vi "LD-Cal-CircleCenterXY -矩形.vi"(0 "Image in":T5(plugin-control), 5 "String":string=";1480.000;1115.000;378.000;757.000;0.000;0.000;0;1;3;3;10.000;4;0;1;0;0;1;65280;255;16776960;16711680;;3;10;3;23;255", 11 "error in":errorcluster) -> (4 "Image Out":T5(plugin-control), 6 "Straight Edge (Find Straight Edge 2)":T4 {"Point2 (Real-World)"."Y" format="%.2f"; "Point2 (Real-World)"."X" format="%.2f"; "Point1 (Real-World)"."Y" format="%.2f"; "Point1 (Real-World)"."X" format="%.2f"; "Point2 (Pixels)"."Y" format="%.2f"; "Point2 (Pixels)"."X" format="%.2f"; "Point1 (Pixels)"."Y" format="%.2f"; "Point1 (Pixels)"."X" format="%.2f"}, 8 "Angle (Pixel)":dbl, 10 "result string":string, 15 "error out":errorcluster)   [LabVIEW 2015]
uses:
  <vilib>/vision/Measure.llb/Edge Options.ctl
  <vilib>/vision/Measure.llb/Edge Polarity.ctl
  <vilib>/vision/Measure.llb/Straight Edge Options.ctl
  <vilib>/vision/Measure.llb/Straight Edge Process.ctl
panel:
  out "Angle (Pixel) 3":dbl
  in  "Options (Find Straight Edge 2)":T3={"Search Direction"=2, "Edge Options"={"Edge Polarity"=2, "Kernel Size"=5, "Width"=11, "Minimum Edge Strength"=76.237114, "Interpolation Type"=enum."Bilinear Fixed", "Data Processing Method"=enum."Average"}, "Show Search Area"=TRUE, "Show Search Lines"=TRUE, "Show Edges Found"=TRUE, "Show Result"=TRUE, "Search Area Color"=65280, "Search Lines Color"=255, "Edge Locations Color"=16776960, "Result Color"=16711680, "Overlay Group Name"=""} {"Search Direction" items=["Left to Right", "Right to Left", "Top to Bottom", "Bottom to Top"]; "Edge Options"."Edge Polarity" items=["All Edges", "Rising Edges", "Falling Edges"]; "Edge Options"."Minimum Edge Strength" format="%.2f"; "Edge Options"."Width" step=2; "Edge Options"."Kernel Size" step=2}
  in  "Option All":T3 {"Edge Options"."Edge Polarity" items=["All Edges", "Rising Edges", "Falling Edges"]; "Edge Options"."Minimum Edge Strength" format="%.2f"; "Edge Options"."Width" step=2; "Edge Options"."Kernel Size" step=2}
  out "Center (Pixels)":cluster{"X":string, "Y":string, "Radius":string}
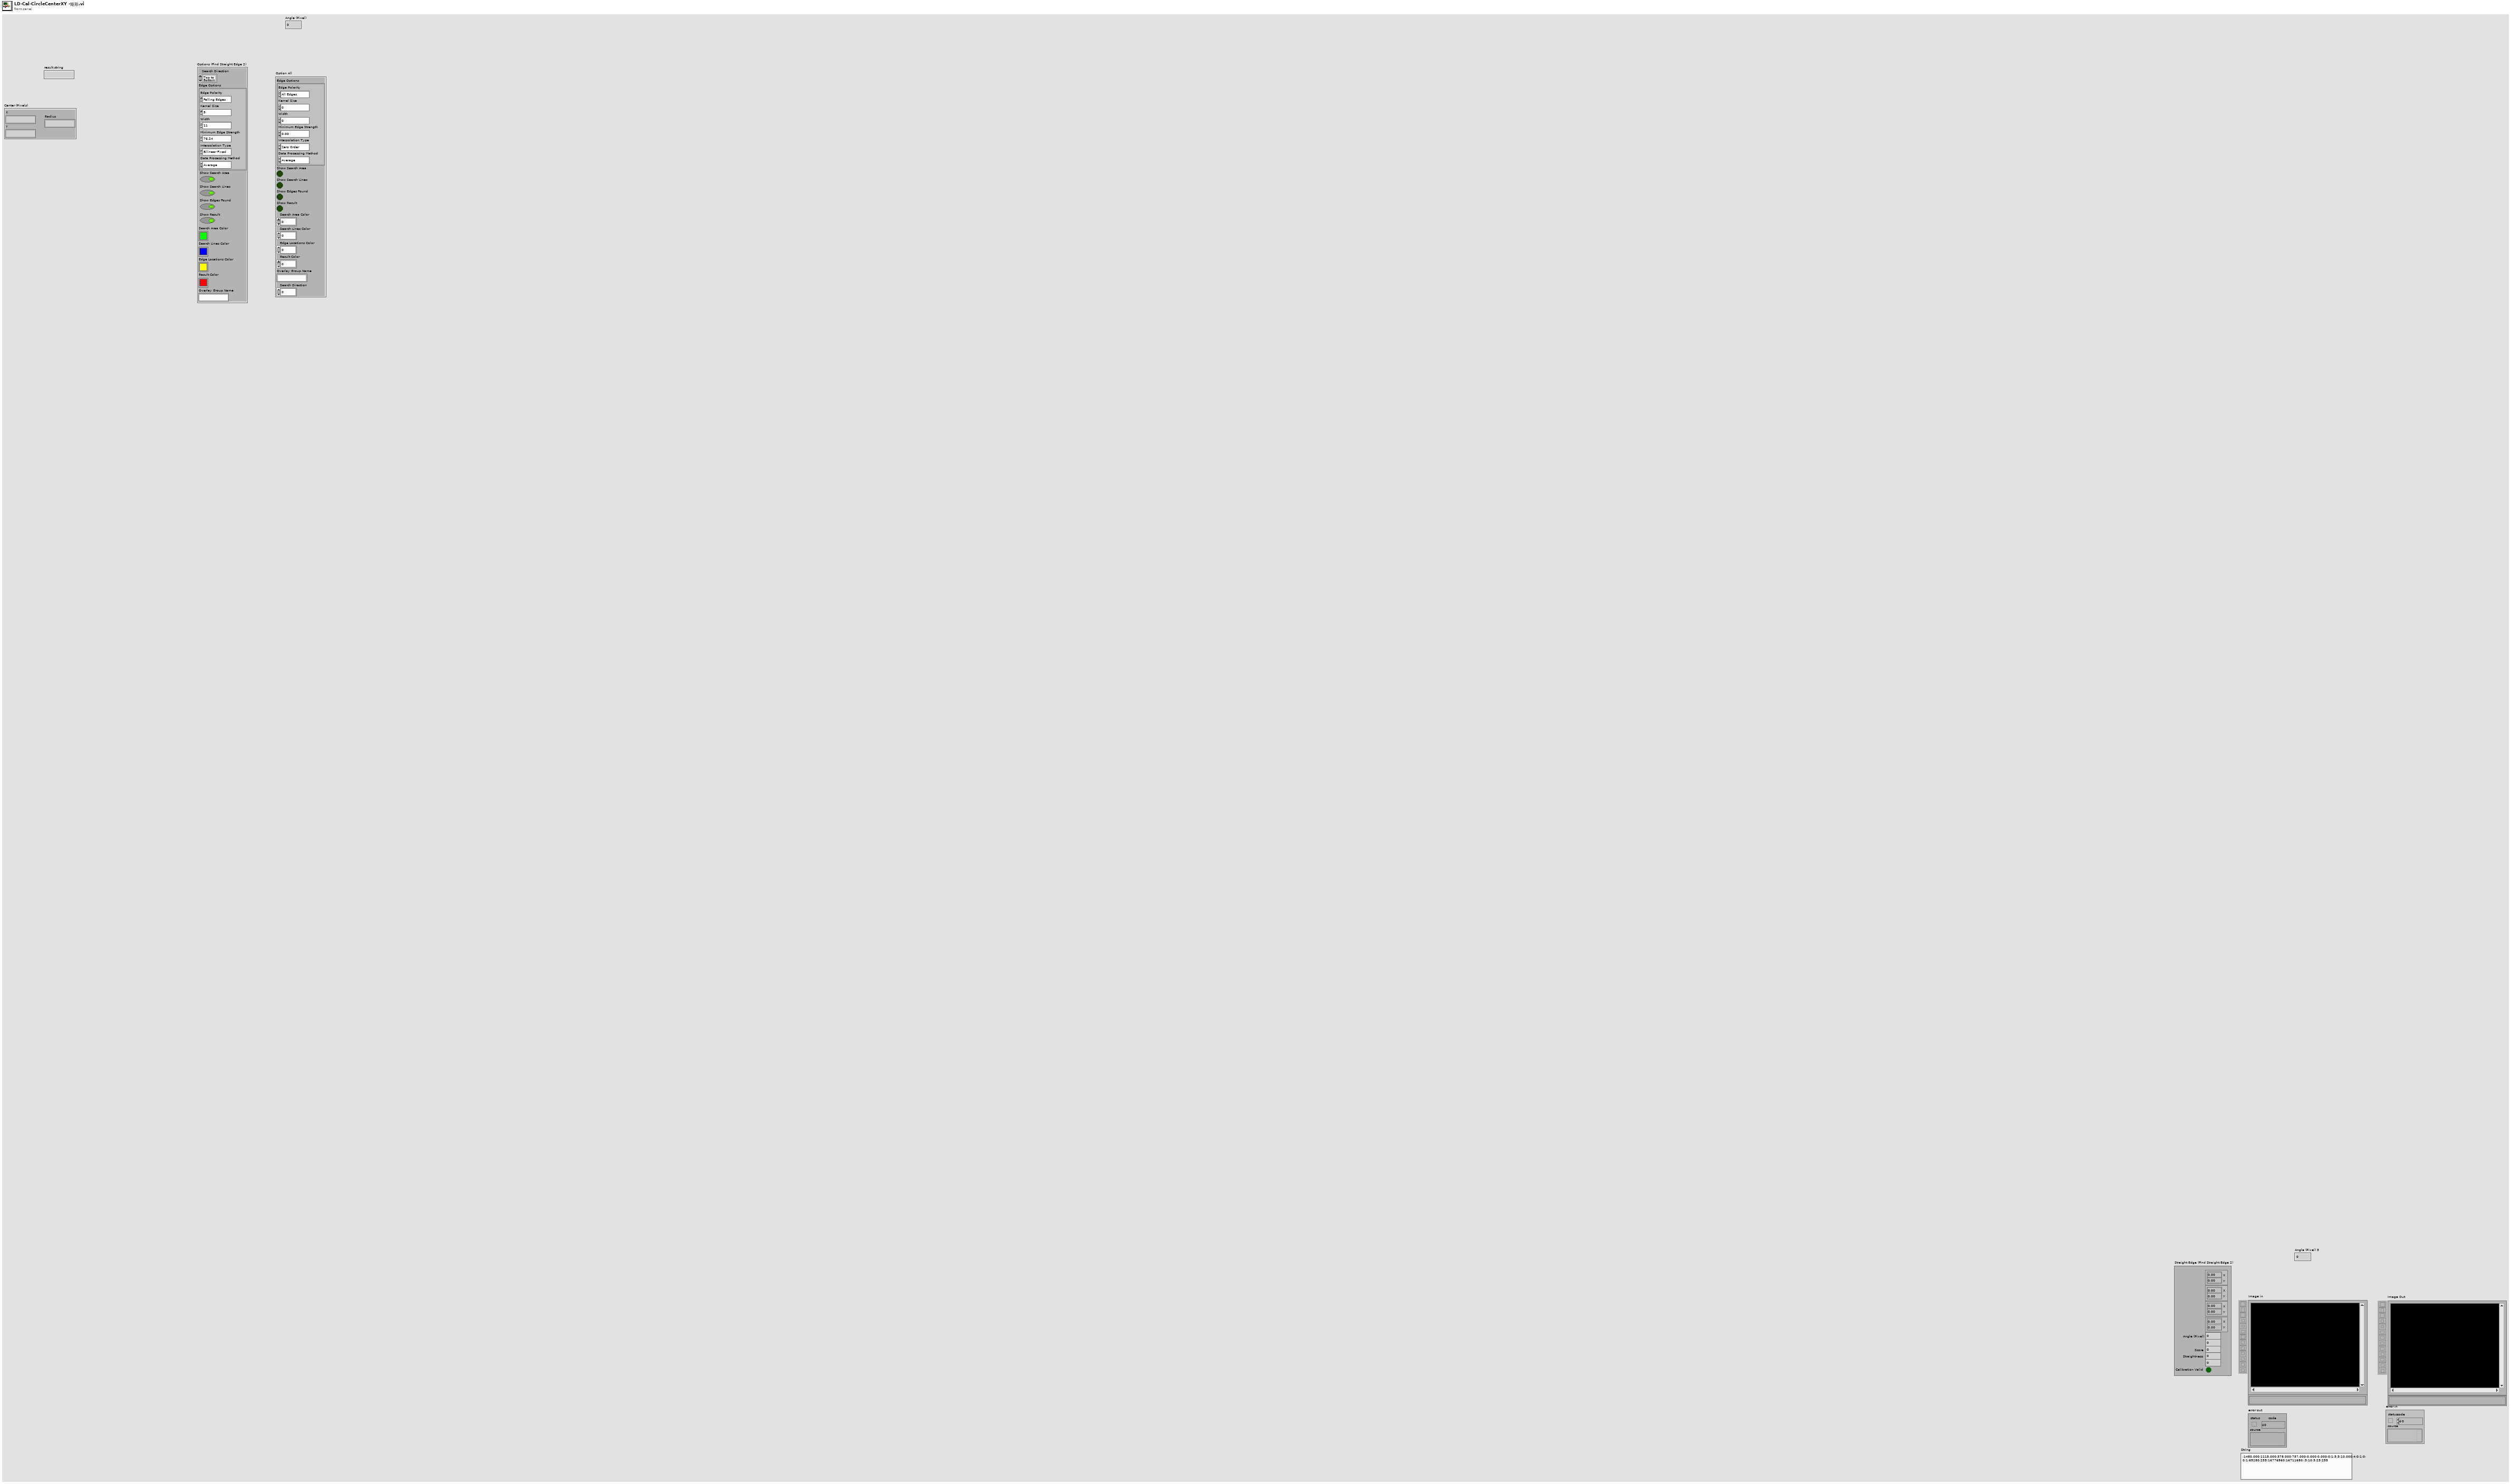
[diagram p1: front panel]
types:
  T1 = typedef "Edge Options.ctl" = cluster{"Edge Polarity":T2, "Kernel Size":u32, "Width":u32, "Minimum Edge Strength":sgl, "Interpolation Type":enum32{"Zero Order", "Bilinear", "Quadratic", "Cubic", "Bilinear Fixed"}, "Data Processing Method":enum32{"Average", "Median"}}
  T2 = typedef "Edge Polarity.ctl" = u32
  T3 = cluster{"Search Direction":u32, "Edge Options":T1, "Show Search Area":bool, "Show Search Lines":bool, "Show Edges Found":bool, "Show Result":bool, "Search Area Color":u32, "Search Lines Color":u32, "Edge Locations Color":u32, "Result Color":u32, "Overlay Group Name":string}
  T4 = cluster{"Point1 (Pixels)":cluster{"X":sgl, "Y":sgl}, "Point2 (Pixels)":cluster{"X":sgl, "Y":sgl}, "Point1 (Real-World)":cluster{"X":sgl, "Y":sgl}, "Point2 (Real-World)":cluster{"X":sgl, "Y":sgl}, "Angle (Pixel)":dbl, "Angle (Real-World)":dbl, "Score":dbl, "Straightness":dbl, "Average SNR (db)":dbl, "Calibration Valid":bool}
  T5 = typedef "IMAQ Image.ctl" = refnum<image>
  T6 = typedef "Straight Edge Options.ctl" = cluster{"Number of Lines":i32, "Type":T7, "Min. Score":dbl, "Max. Score":dbl, "Orientation":dbl, "Angle Range":dbl, "Angle Tolerance":dbl, "Step Size":u32, "Min. SNR (db)":dbl, "Min. Points (%)":dbl, "Hough Iterations":i32}
  T7 = typedef "Straight Edge Process.ctl" = enum32{"First Edge Rake", "Best Edge Rake", "Hough Edge Rake", "First Edge Projection", "Best Edge Projection"}
  T8 = typedef "Image Type" = u32
  T9 = typedef "ROI Descriptor" = cluster{"Global Rectangle":i32[], "Contours":cluster{"ID":enum32{"External", "Internal"}, "Type":u32, "Coordinates":i32[]}[]}
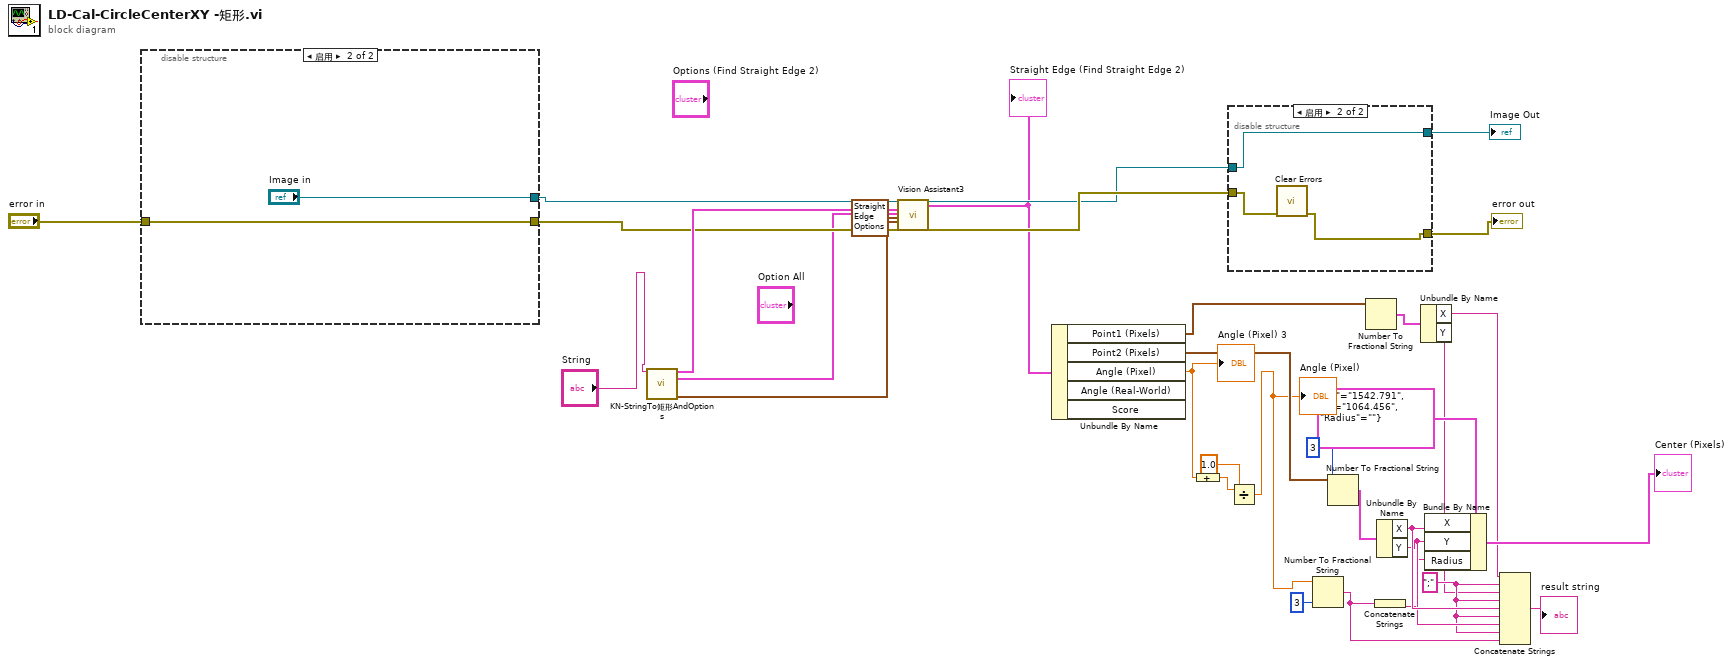
[diagram p0: block diagram]
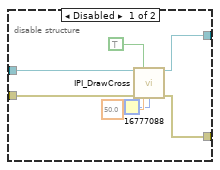
[diagram p2: hidden frame]
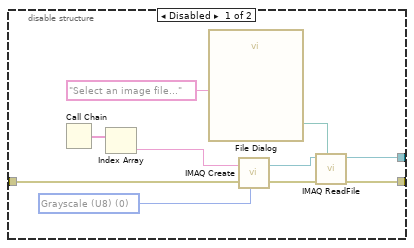
[diagram p3: hidden frame]
diagram:
  w2 = ";" ("字符串")
  n1 = disable-structure shown="启用" {
    disable-tunnel: "error in" -> [w41 w45]
    disable-tunnel: [w35 "Image in"] -> w29
    disable-tunnel: [w34 w45] -> w26
    frame Disabled {
      w36 = T8 0 items=["Grayscale (U8)", "Grayscale (I16)", "Grayscale (SGL)", "Complex (CSG)", "RGB (U32)", "HSL (U32)", "RGB (U64)", "Grayscale (U16)"] ("Image Type")
      n2 = Call Chain() -> (call chain=w40:string[])
      n3 = Index Array(array=w40) -> (element=w39:string)  [unwired: 1 in]
      n4 = call "File Dialog"("prompt"="Select an image file...") -> ("selected path"=w37:path)  [unwired: 6 in, 8 out]
      n5 = call "IMAQ Create"("Image Name"=w39, "Image Type"=w36, "error in (no error)"=w41) -> ("New Image"=w43:T5, "error out"=w42:errorcluster)  [unwired: 1 in, 1 out]
      n6 = call "IMAQ ReadFile"("File Path"=w37, "error in (no error)"=w42, "Image"=w43) -> ("error out"=w34:errorcluster, "Image Out"=w35:T5)  [unwired: 2 in, 5 out]
    }
    frame Enabled {
    }
  }
  n7 = call "KN-StringTo矩形AndOptions.vi"("String"="String") -> ("ROI Descriptor"=w28:T9, "Option All"=w11:T3, "Range (Threshold 1)"=w27:cluster{"Lower value":sgl, "Upper value":sgl})  [unwired: 11 in, 1 out]
  n8 = call "Vision Assistant3"("Image In"=w29, "ROI Descriptor (Find Straight Edge 2)"=w28, "Options (Find Straight Edge 2)"=w11, "Fit Options (Find Straight Edge 2)"=T6 {"Number of Lines"=1, "Type"=enum."Best Edge Rake", "Min. Score"=10.0, "Max. Score"=1000.0, "Orientation"=0.0, "Angle Range"=45.0, "Angle Tolerance"=1.0, "Step Size"=17, "Min. SNR (db)"=0.0, "Min. Points (%)"=25.0, "Hough Iterations"=5}, "Range (Threshold 1)"=w27, "error in"=w26) -> ("Image Out"=w24:T5, "Straight Edge (Find Straight Edge 2)"=w12:T4, "error out"=w25:errorcluster)  [unwired: 19 in]
  "Straight Edge (Find Straight Edge 2)" <- w12
  n9 = Unbundle By Name(w12) -> ("Point1 (Pixels)"=w5:cluster{"X":sgl, "Y":sgl}, "Point2 (Pixels)"=w23:cluster{"X":sgl, "Y":sgl}, "Angle (Pixel)"=w7:dbl)  [unwired: 2 out]
  "Angle (Pixel) 3" <- w7
  n10 = Compound Arithmetic op=ADD(w7) -> (w9:dbl)
  n11 = disable-structure shown="启用" {
    disable-tunnel: w24 -> [w54 w57]
    disable-tunnel: [w53 w57] -> w32
    disable-tunnel: w25 -> [w47 w56]
    disable-tunnel: [w46 w55] -> w31
    frame Disabled {
      n12 = call "IPI_DrawCross.vi"("Image In"=w54, "Show Cross"=TRUE, "error in (no error)"=w47, "Radius"=50.0, "颜色盒"=u32 16777088) -> ("Image Out"=w53:T5, "X"=w52:dbl, "Y"=w51:dbl, "error out"=w46:errorcluster)  [unwired: 7 in]
    }
    frame Enabled {
      n13 = call <vilib>:"Clear Errors.vi"("error in (no error)"=w56) -> ("error out"=w55:errorcluster)  [unwired: 5 in, 1 out]
    }
  }
  "error out" <- w31
  "Image Out" <- w32
  n14 = Divide(x=w9, y=1.0) -> (x/y=w6:dbl)
  "Angle (Pixel)" <- w6
  n15 = Number To Fractional String(number=w6, precision (6)=i16 3 ("精度(6)")) -> (F-format string=w14:string)  [unwired: 2 in]
  n16 = Number To Fractional String(number=w23, precision (6)=i16 3 ("精度(6)")) -> (F-format string=w19:cluster{"X":string, "Y":string})  [unwired: 2 in]
  n17 = Number To Fractional String(number=w5) -> (F-format string=w4:cluster{"X":string, "Y":string})  [unwired: 3 in]
  n18 = Concatenate Strings(w14) -> (w13:string)
  n19 = Unbundle By Name(w19) -> ("X"=w17:string, "Y"=w16:string)
  n20 = Unbundle By Name(w4) -> ("X"=w3:string, "Y"=w1:string)
  n21 = Bundle By Name(cluster=cluster{"X":string, "Y":string, "Radius":string} {"X"="1542.791", "Y"="1064.456", "Radius"=""} ("Center (Pixels) 2"), "X"=w17, "Y"=w16, "Radius"=w13) -> (→"Center (Pixels)":cluster{"X":string, "Y":string, "Radius":string})
  n22 = Concatenate Strings(w3, w2, w1, w2, w17, w2, w16, w2, w14) -> (→"result string":string)
